vi "Version_2.0_Single_Column_Code.vi"() -> ()   [LabVIEW 2020] (continued)
                                n2523 = case shown="\"Standard Pumping\", Default" w2963 {
                                tunnel: w2965 -> [w2970 w2979]
                                tunnel: w2961 -> [w2971 w2978]
                                tunnel: [w2969 w2976] -> w2960
                                tunnel: w2962 -> [w2968 w2977]
                                frame "Standard Pumping", Default {
                                n2524 = Subtract(x=w2970, y=w2971) -> (x-y=w2967:dbl)
                                n2525 = Absolute Value(x=w2967) -> (abs(x)=w2966:dbl)
                                n2526 = Multiply(x=w2966, y=w2968) -> (x*y=w2973:dbl)
                                n2527 = Divide(x=w2973, y=3000.0) -> (x/y=w2969:dbl)
                                }
                                frame "High Resolution Pumping" {
                                n2528 = Subtract(x=w2979, y=w2978) -> (x-y=w2975:dbl)
                                n2529 = Absolute Value(x=w2975) -> (abs(x)=w2974:dbl)
                                n2530 = Multiply(x=w2974, y=w2977) -> (x*y=w2981:dbl)
                                n2531 = Divide(x=w2981, y=24000.0) -> (x/y=w2976:dbl)
                                }
                                }
                                n2532 = local write "Volume being Injected \nin this process"(w2960) -> ()
                                }
                                frame #1 {
                                n2533 = local read "Stopper that ends \nthe main loops"() -> (w2982:bool)
                                n2534 = call "LSPOneStatus (SubVI).vi"("VISA Refnum in"=w2985) -> ("read buffer"=w2987:string)  [unwired: 10 in]
                                n2535 = call <vilib>:"Trim Whitespace.vi"("string"=w2987) -> ("trimmed string"=w2986:string)  [unwired: 1 in]
                                n2536 = Equal?(x=w2986, y="/0`\u0003") -> (x = y?=w2984:bool)
                                n2537 = Or(x=w2984, y=w2982) -> (x .or. y?=w2983:bool)
                                }
                                }
                                n2538 = Wait (ms)(milliseconds to wait=u32 100) -> ()  [unwired: 1 out]
                                n2539 = local read "Stopper that ends \nthe main loops"() -> (w2952:bool)
                                n2540 = case shown="True" w2952 {
                                frame False {
                                }
                                frame True {
                                n2541 = local read "VISA Refnum in\nfor Pump"() -> (w2959:refnum<visa-resource-name>)
                                n2542 = call "HardStopCurrentProcess (SubVI).vi"("VISA Refnum in"=w2959) -> ()  [unwired: 11 in]
                                }
                                }
                                }
                                }
                                frame #11 {
                                # "Change the pump port back to Buffer-C1"
                                n2543 = local read "VISA Refnum in\nfor Pump"() -> (w2990:refnum<visa-resource-name>)
                                n2544 = local read "Port for \nC1-Equilibriation"() -> (w2989:string)
                                n2545 = local write "Pause Data Collection"(TRUE ("Pause Data Collection")) -> ()
                                n2546 = Wait (ms)(milliseconds to wait=u32 500) -> ()  [unwired: 1 out]
                                n2547 = call "PortChanger (SubVI).vi"("Port Number"=w2989, "VISA Refnum in"=w2990) -> ()  [unwired: 10 in]
                                }
                                frame #12 {
                                n2548 = local read "VISA Refnum in\nfor Pump"() -> (w2993:refnum<visa-resource-name>)
                                n2549 = local write "Volume being Injected \nin this process"(0.0 ("Volume being Injected \nin this process")) -> ()
                                n2550 = call "ProcessCompletionWaiter (SubVI).vi"("VISA Refnum in"=w2993) -> ()  [unwired: 11 in]
                                }
                              }
                            }
                            n2551 = local write "Reminder of the \nVolume to be \nPumped"(w2856) -> ()
                          }
                          frame #9 {
                            n2552 = stacked-sequence {
                              frame #0 {
                                n2553 = local read "Buffer-C1 PickUp \nFlow Rate (ul/min)\nfor Equilibration \nof Column-2"() -> (w2997:dbl)
                                n2554 = local read "Buffer-C1 Pumping\nResolution \nfor Equilibration \nof Column-2"() -> (w2996:T2)
                                n2555 = local read "VISA Refnum in\nfor Pump"() -> (w2999:refnum<visa-resource-name>)
                                n2556 = local read "Reminder of the \nVolume to be \nPumped"() -> (w2995:dbl)
                                n2557 = local read "Volume of Syringe"() -> (w2998:dbl)
                                n2558 = call "RPickUp(SubVI).vi"("Volume to be picked up"=w2995, "Volume of Syringe"=w2998, "Resolution of PickUP"=w2996, "PickUp Flow Rate (ul/min)"=w2997, "VISA Refnum in"=w2999) -> ()  [unwired: 6 in, 1 out]
                              }
                              frame #1 {
                                n2559 = while {
                                stop <- w3000 stop-if-true
                                n2560 = local read "Stopper that ends \nthe main loops"() -> (w3001:bool)
                                n2561 = local read "VISA Refnum in\nfor Pump"() -> (w3002:refnum<visa-resource-name>)
                                n2562 = case shown="True" w3001 {
                                frame False {
                                }
                                frame True {
                                n2563 = local read "VISA Refnum in\nfor Pump"() -> (w3003:refnum<visa-resource-name>)
                                n2564 = call "HardStopCurrentProcess (SubVI).vi"("VISA Refnum in"=w3003) -> ()  [unwired: 11 in]
                                }
                                }
                                n2565 = call "ProcessCompletionWaiterWithOutPut (SubVI).vi"("VISA Refnum in"=w3002) -> ("Boolean"=w3000:bool)  [unwired: 10 in]
                                }
                              }
                              frame #2 {
                                # "Reads the initial Plunger Position for computing the volume dispensed"
                                n2566 = local read "VISA Refnum in\nfor Pump"() -> (w3005:refnum<visa-resource-name>)
                                n2567 = call "AbsolutePlungerPosition (SubVI).vi"("VISA Refnum in"=w3005) -> ("Plunger Position"=w3004:i32)  [unwired: 10 in]
                                n2568 = local write "Initial Plunger Position"(w3004) -> ()
                              }
                              frame #3 {
                                # "Switch to Port-10"
                                # "Port-10 of the pump is conncted to column-2 of chip"
                                n2569 = local read "VISA Refnum in\nfor Pump"() -> (w3007:refnum<visa-resource-name>)
                                n2570 = call "PortChanger (SubVI).vi"("Port Number"="10", "VISA Refnum in"=w3007) -> ()  [unwired: 10 in]
                              }
                              frame #4 {
                                n2571 = while {
                                stop <- w3008 stop-if-true
                                n2572 = local read "Stopper that ends \nthe main loops"() -> (w3009:bool)
                                n2573 = local read "VISA Refnum in\nfor Pump"() -> (w3010:refnum<visa-resource-name>)
                                n2574 = case shown="True" w3009 {
                                frame False {
                                }
                                frame True {
                                n2575 = local read "VISA Refnum in\nfor Pump"() -> (w3011:refnum<visa-resource-name>)
                                n2576 = call "HardStopCurrentProcess (SubVI).vi"("VISA Refnum in"=w3011) -> ()  [unwired: 11 in]
                                }
                                }
                                n2577 = call "ProcessCompletionWaiterWithOutPut (SubVI).vi"("VISA Refnum in"=w3010) -> ("Boolean"=w3008:bool)  [unwired: 10 in]
                                }
                              }
                              frame #5 {
                                # "Keeps the AMF valve after column-1 open and valve after column-2 closed"
                                n2578 = local read "Buffer-C1 Dispense\nFlow Rate (ul/min) \nfor Equilibration\nof Column-2"() -> (w3024:dbl)
                                n2579 = local read "Buffer-C1 Pumping\nResolution \nfor Equilibration \nof Column-2"() -> (w3023:T2)
                                n2580 = local read "VISA Refnum in\nfor Pump"() -> (w3026:refnum<visa-resource-name>)
                                n2581 = local write "Pause Data Collection"(FALSE ("Pause Data Collection")) -> ()
                                n2582 = local read "Volume of Syringe"() -> (w3025:dbl)
                                n2583 = call "GoToAbsolutePosition(SubVI).vi"("Absolute Volume Position in Syringe (in ul)"=0.0, "Volume of Syringe"=w3025, "Resolution of Pumping"=w3023, "Flow Rate (ul/min)"=w3024, "VISA Refnum in"=w3026) -> ()  [unwired: 6 in, 1 out]
                                n2584 = local read "VISA Refnum in\nfor Valve"() -> (w3016:refnum<visa-resource-name>)
                                n2585 = local write "Valve V1 Open"(FALSE ("Valve V1 Open")) -> ()
                                n2586 = local write "Valve V2 Open"(TRUE ("Valve V2 Open")) -> ()
                                n2587 = local write "Valve V3 Open"(TRUE ("Valve V3 Open")) -> ()
                                n2588 = local write "Valve V4 Open"(FALSE ("Affinity On")) -> ()
                                n2589 = local read "External Valve \nOPEN"() -> (w3015:string)
                                n2590 = local write "Valve V5 Open"(FALSE ("Valve V5 Open")) -> ()
                                n2591 = local write "Valve V6 Open"(FALSE ("Valve V6 Open")) -> ()
                                n2592 = local write "Valve V7 Open"(FALSE ("Valve V7 Open")) -> ()
                                n2593 = call "PortChanger_Valve (SubVI).vi"("Port Number"=w3015, "VISA Refnum in"=w3016) -> ()  [unwired: 10 in]
                              }
                              frame #6 {
                                n2594 = local read "Buffer-C1 Pumping\nResolution \nfor Equilibration \nof Column-2"() -> (w3028:T2)
                                n2595 = local read "VISA Refnum in\nfor Pump"() -> (w3030:refnum<visa-resource-name>)
                                n2596 = local read "Initial Plunger Position"() -> (w3029:dbl)
                                n2597 = local read "Volume of Syringe"() -> (w3027:dbl)
                                n2598 = while {
                                tunnel: w3029 -> [w3037]
                                tunnel: w3030 -> [w3036]
                                tunnel: w3028 -> [w3035]
                                tunnel: w3027 -> [w3034]
                                stop <- w3032 stop-if-true
                                n2599 = stacked-sequence {
                                tunnel: w3037 -> [w3044 _]
                                tunnel: w3036 -> [w3043 w3068]
                                tunnel: w3035 -> [w3042 _]
                                tunnel: w3034 -> [w3041 _]
                                tunnel: [_ w3066] -> w3032
                                frame #0 {
                                n2600 = call "AbsolutePlungerPosition (SubVI).vi"("VISA Refnum in"=w3043) -> ("Plunger Position"=w3040:i32)  [unwired: 10 in]
                                n2601 = case shown="\"Standard Pumping\", Default" w3042 {
                                tunnel: w3044 -> [w3049 w3058]
                                tunnel: w3040 -> [w3050 w3057]
                                tunnel: [w3048 w3055] -> w3039
                                tunnel: w3041 -> [w3047 w3056]
                                frame "Standard Pumping", Default {
                                n2602 = Subtract(x=w3049, y=w3050) -> (x-y=w3046:dbl)
                                n2603 = Absolute Value(x=w3046) -> (abs(x)=w3045:dbl)
                                n2604 = Multiply(x=w3045, y=w3047) -> (x*y=w3052:dbl)
                                n2605 = Divide(x=w3052, y=3000.0) -> (x/y=w3048:dbl)
                                }
                                frame "High Resolution Pumping" {
                                n2606 = Subtract(x=w3058, y=w3057) -> (x-y=w3054:dbl)
                                n2607 = Absolute Value(x=w3054) -> (abs(x)=w3053:dbl)
                                n2608 = Multiply(x=w3053, y=w3056) -> (x*y=w3060:dbl)
                                n2609 = Divide(x=w3060, y=24000.0) -> (x/y=w3055:dbl)
                                }
                                }
                                n2610 = local write "Volume being Injected \nin this process"(w3039) -> ()
                                }
                                frame #1 {
                                n2611 = local read "Buffer-C Volume \nto be Pumped for\nColumn \nnon-interference"() -> (w3064:dbl)
                                n2612 = local read "Volume being Injected \nin this process"() -> (w3065:dbl)
                                n2613 = local read "Stopper that ends \nthe main loops"() -> (w3063:bool)
                                n2614 = call "LSPOneStatus (SubVI).vi"("VISA Refnum in"=w3068) -> ("read buffer"=w3070:string)  [unwired: 10 in]
                                n2615 = call <vilib>:"Trim Whitespace.vi"("string"=w3070) -> ("trimmed string"=w3069:string)  [unwired: 1 in]
                                n2616 = Equal?(x=w3069, y="/0`\u0003") -> (x = y?=w3067:bool)
                                n2617 = Greater Or Equal?(x=w3065, y=w3064) -> (x >= y?=w3062:bool)
                                n2618 = Or(x=w3063, y=w3062) -> (x .or. y?=w3061:bool)
                                n2619 = Or(x=w3067, y=w3061) -> (x .or. y?=w3066:bool)
                                }
                                }
                                n2620 = Wait (ms)(milliseconds to wait=u32 100) -> ()  [unwired: 1 out]
                                n2621 = local read "Stopper that ends \nthe main loops"() -> (w3031:bool)
                                n2622 = case shown="True" w3031 {
                                frame False {
                                }
                                frame True {
                                n2623 = local read "VISA Refnum in\nfor Pump"() -> (w3038:refnum<visa-resource-name>)
                                n2624 = call "HardStopCurrentProcess (SubVI).vi"("VISA Refnum in"=w3038) -> ()  [unwired: 11 in]
                                }
                                }
                                }
                              }
                              frame #7 {
                                # "Keeps the AMF valve after column-1 closed and valve after column-2 open"
                                n2625 = local read "VISA Refnum in\nfor Valve"() -> (w3076:refnum<visa-resource-name>)
                                n2626 = local read "External Valve \nCLOSED"() -> (w3075:string)
                                n2627 = local write "Valve V4 Open"(TRUE ("Valve V4 Open")) -> ()
                                n2628 = local write "Valve V1 Open"(FALSE ("Valve V1 Open")) -> ()
                                n2629 = local write "Valve V2 Open"(FALSE ("Valve V2 Open")) -> ()
                                n2630 = local write "Valve V3 Open"(FALSE ("Valve V3 Open")) -> ()
                                n2631 = call "PortChanger_Valve (SubVI).vi"("Port Number"=w3075, "VISA Refnum in"=w3076) -> ()  [unwired: 10 in]
                                n2632 = local write "Valve V7 Open"(TRUE ("Valve V7 Open")) -> ()
                                n2633 = local write "Valve V5 Open"(TRUE ("Valve V5 Open")) -> ()
                                n2634 = local write "Valve V6 Open"(TRUE ("Valve V6 Open")) -> ()
                              }
                              frame #8 {
                                n2635 = local read "Buffer-C1 Pumping\nResolution \nfor Equilibration \nof Column-2"() -> (w3082:T2)
                                n2636 = local read "VISA Refnum in\nfor Pump"() -> (w3084:refnum<visa-resource-name>)
                                n2637 = local read "Initial Plunger Position"() -> (w3083:dbl)
                                n2638 = local read "Volume of Syringe"() -> (w3081:dbl)
                                n2639 = while {
                                tunnel: w3083 -> [w3091]
                                tunnel: w3084 -> [w3090]
                                tunnel: w3082 -> [w3089]
                                tunnel: w3081 -> [w3088]
                                stop <- w3086 stop-if-true
                                n2640 = stacked-sequence {
                                tunnel: w3091 -> [w3098 _]
                                tunnel: w3090 -> [w3097 w3118]
                                tunnel: w3089 -> [w3096 _]
                                tunnel: w3088 -> [w3095 _]
                                tunnel: [_ w3116] -> w3086
                                frame #0 {
                                n2641 = call "AbsolutePlungerPosition (SubVI).vi"("VISA Refnum in"=w3097) -> ("Plunger Position"=w3094:i32)  [unwired: 10 in]
                                n2642 = case shown="\"Standard Pumping\", Default" w3096 {
                                tunnel: w3098 -> [w3103 w3112]
                                tunnel: w3094 -> [w3104 w3111]
                                tunnel: [w3102 w3109] -> w3093
                                tunnel: w3095 -> [w3101 w3110]
                                frame "Standard Pumping", Default {
                                n2643 = Subtract(x=w3103, y=w3104) -> (x-y=w3100:dbl)
                                n2644 = Absolute Value(x=w3100) -> (abs(x)=w3099:dbl)
                                n2645 = Multiply(x=w3099, y=w3101) -> (x*y=w3106:dbl)
                                n2646 = Divide(x=w3106, y=3000.0) -> (x/y=w3102:dbl)
                                }
                                frame "High Resolution Pumping" {
                                n2647 = Subtract(x=w3112, y=w3111) -> (x-y=w3108:dbl)
                                n2648 = Absolute Value(x=w3108) -> (abs(x)=w3107:dbl)
                                n2649 = Multiply(x=w3107, y=w3110) -> (x*y=w3114:dbl)
                                n2650 = Divide(x=w3114, y=24000.0) -> (x/y=w3109:dbl)
                                }
                                }
                                n2651 = local write "Volume being Injected \nin this process"(w3093) -> ()
                                }
                                frame #1 {
                                n2652 = local read "Stopper that ends \nthe main loops"() -> (w3115:bool)
                                n2653 = call "LSPOneStatus (SubVI).vi"("VISA Refnum in"=w3118) -> ("read buffer"=w3120:string)  [unwired: 10 in]
                                n2654 = call <vilib>:"Trim Whitespace.vi"("string"=w3120) -> ("trimmed string"=w3119:string)  [unwired: 1 in]
                                n2655 = Equal?(x=w3119, y="/0`\u0003") -> (x = y?=w3117:bool)
                                n2656 = Or(x=w3117, y=w3115) -> (x .or. y?=w3116:bool)
                                }
                                }
                                n2657 = Wait (ms)(milliseconds to wait=u32 100) -> ()  [unwired: 1 out]
                                n2658 = local read "Stopper that ends \nthe main loops"() -> (w3085:bool)
                                n2659 = case shown="True" w3085 {
                                frame False {
                                }
                                frame True {
                                n2660 = local read "VISA Refnum in\nfor Pump"() -> (w3092:refnum<visa-resource-name>)
                                n2661 = call "HardStopCurrentProcess (SubVI).vi"("VISA Refnum in"=w3092) -> ()  [unwired: 11 in]
                                }
                                }
                                }
                              }
                              frame #9 {
                                n2662 = local write "Pause Data Collection"(TRUE ("Pause Data Collection")) -> ()
                                n2663 = Wait (ms)(milliseconds to wait=u32 500) -> ()  [unwired: 1 out]
                              }
                              frame #10 {
                                n2664 = local write "Volume being Injected \nin this process"(0.0 ("Volume being Injected \nin this process")) -> ()
                                n2665 = local write "Start the Process"(FALSE ("Start the Process")) -> ()
                              }
                            }
                          }
                          frame #10 {
                            # "Clean the tubing with Sample"
                            n2666 = local read "N-S"() -> (w3126:i32)
                            n2667 = for {
                              N: w3126 -> [_]
                              n2668 = stacked-sequence {
                                frame #0 {
                                n2669 = local read "VISA Refnum in\nfor Pump"() -> (w3129:refnum<visa-resource-name>)
                                n2670 = local read "Port for \nSample"() -> (w3128:string)
                                n2671 = call "PortChanger (SubVI).vi"("Port Number"=w3128, "VISA Refnum in"=w3129) -> ()  [unwired: 10 in]
                                }
                                frame #1 {
                                n2672 = local read "VISA Refnum in\nfor Pump"() -> (w3130:refnum<visa-resource-name>)
                                n2673 = call "ProcessCompletionWaiter (SubVI).vi"("VISA Refnum in"=w3130) -> ()  [unwired: 11 in]
                                }
                                frame #2 {
                                n2674 = local read "VISA Refnum in\nfor Pump"() -> (w3135:refnum<visa-resource-name>)
                                n2675 = local read "Sample PickUp \nFlow Rate (ul/min)"() -> (w3132:dbl)
                                n2676 = local read "V-S"() -> (w3131:dbl)
                                n2677 = local read "Volume of Syringe"() -> (w3133:dbl)
                                n2678 = call "RPickUp(SubVI).vi"("Volume to be picked up"=w3131, "Volume of Syringe"=w3133, "Resolution of PickUP"=T2."Standard Pumping", "PickUp Flow Rate (ul/min)"=w3132, "VISA Refnum in"=w3135) -> ()  [unwired: 6 in, 1 out]
                                }
                                frame #3 {
                                n2679 = local read "Stopper that ends \nthe main loops"() -> (w3136:bool)
                                n2680 = local read "VISA Refnum in\nfor Pump"() -> (w3137:refnum<visa-resource-name>)
                                n2681 = case shown="True" w3136 {
                                frame False {
                                }
                                frame True {
                                n2682 = local read "VISA Refnum in\nfor Pump"() -> (w3138:refnum<visa-resource-name>)
                                n2683 = call "HardStopCurrentProcess (SubVI).vi"("VISA Refnum in"=w3138) -> ()  [unwired: 11 in]
                                }
                                }
                                n2684 = call "ProcessCompletionWaiter (SubVI).vi"("VISA Refnum in"=w3137) -> ()  [unwired: 11 in]
                                }
                                frame #4 {
                                n2685 = local read "VISA Refnum in\nfor Pump"() -> (w3140:refnum<visa-resource-name>)
                                n2686 = call "PortChanger (SubVI).vi"("Port Number"="1", "VISA Refnum in"=w3140) -> ()  [unwired: 10 in]
                                }
                                frame #5 {
                                n2687 = local read "Stopper that ends \nthe main loops"() -> (w3141:bool)
                                n2688 = local read "VISA Refnum in\nfor Pump"() -> (w3142:refnum<visa-resource-name>)
                                n2689 = case shown="True" w3141 {
                                frame False {
                                }
                                frame True {
                                n2690 = local read "VISA Refnum in\nfor Pump"() -> (w3143:refnum<visa-resource-name>)
                                n2691 = call "HardStopCurrentProcess (SubVI).vi"("VISA Refnum in"=w3143) -> ()  [unwired: 11 in]
                                }
                                }
                                n2692 = call "ProcessCompletionWaiter (SubVI).vi"("VISA Refnum in"=w3142) -> ()  [unwired: 11 in]
                                }
                                frame #6 {
                                n2693 = local read "VISA Refnum in\nfor Pump"() -> (w3148:refnum<visa-resource-name>)
                                n2694 = local read "Volume of Syringe"() -> (w3145:dbl)
                                n2695 = call "GoToAbsolutePosition(SubVI).vi"("Absolute Volume Position in Syringe (in ul)"=0.0 ("Volume to be picked up"), "Volume of Syringe"=w3145, "Resolution of Pumping"=T2."Standard Pumping" ("Resolution of PickUP"), "Flow Rate (ul/min)"=150.0 ("PickUp Flow Rate (ul/min)"), "VISA Refnum in"=w3148) -> ()  [unwired: 6 in, 1 out]
                                }
                                frame #7 {
                                n2696 = local read "Stopper that ends \nthe main loops"() -> (w3149:bool)
                                n2697 = local read "VISA Refnum in\nfor Pump"() -> (w3150:refnum<visa-resource-name>)
                                n2698 = case shown="True" w3149 {
                                frame False {
                                }
                                frame True {
                                n2699 = local read "VISA Refnum in\nfor Pump"() -> (w3151:refnum<visa-resource-name>)
                                n2700 = call "HardStopCurrentProcess (SubVI).vi"("VISA Refnum in"=w3151) -> ()  [unwired: 11 in]
                                }
                                }
                                n2701 = call "ProcessCompletionWaiter (SubVI).vi"("VISA Refnum in"=w3150) -> ()  [unwired: 11 in]
                                }
                              }
                              n2702 = local write "Pause Data Collection"(TRUE ("Pause Data Collection")) -> ()
                            }
                          }
                        }
                      }
                      frame #1 {
                        # "Pump Purified Sample into Column-2"
                        n2703 = stacked-sequence {
                          frame #0 {
                            # "Switch to Port-3"
                            # "Port-3 of pump is connected to Sample"
                            n2704 = local read "VISA Refnum in\nfor Pump"() -> (w3156:refnum<visa-resource-name>)
                            n2705 = local read "Port for \nSample"() -> (w3155:string)
                            n2706 = call "PortChanger (SubVI).vi"("Port Number"=w3155, "VISA Refnum in"=w3156) -> ()  [unwired: 10 in]
                          }
                          frame #1 {
                            n2707 = local read "VISA Refnum in\nfor Pump"() -> (w3157:refnum<visa-resource-name>)
                            n2708 = call "ProcessCompletionWaiter (SubVI).vi"("VISA Refnum in"=w3157) -> ()  [unwired: 11 in]
                          }
                          frame #2 {
                            # "V4 is open"
                            # "V1, V2 and V3 are closed"
                            n2709 = local read "VISA Refnum in\nfor Valve"() -> (w3162:refnum<visa-resource-name>)
                            n2710 = local read "External Valve \nCLOSED"() -> (w3161:string)
                            n2711 = local write "Valve V1 Open"(FALSE ("Valve V1 Open")) -> ()
                            n2712 = local write "Valve V2 Open"(FALSE ("Valve V2 Open")) -> ()
                            n2713 = local write "Valve V3 Open"(FALSE ("Valve V3 Open")) -> ()
                            n2714 = local write "Valve V4 Open"(TRUE ("Valve V4 Open")) -> ()
                            n2715 = call "PortChanger_Valve (SubVI).vi"("Port Number"=w3161, "VISA Refnum in"=w3162) -> ()  [unwired: 10 in]
                            n2716 = local write "Valve V5 Open"(TRUE ("Valve V5 Open")) -> ()
                            n2717 = local write "Valve V6 Open"(TRUE ("Valve V6 Open")) -> ()
                            n2718 = local write "Valve V7 Open"(FALSE ("Valve V7 Open")) -> ()
                          }
                          frame #3 {
                            n2719 = local read "Apparent Volume\nof Syringe"() -> (w3167:dbl)
                            n2720 = local read "Sample Volume \nto be Pumped"() -> (w3170:dbl)
                            n2721 = Quotient & Remainder(x=w3170, y=w3167) -> (x-y*floor(x/y)=w3168:dbl, floor(x/y)=w3169:dbl)
                            n2722 = for {
                              N: w3169 -> [_]
                              n2723 = stacked-sequence {
                                frame #0 {
                                n2724 = local read "Sample PickUp \nFlow Rate (ul/min)"() -> (w3173:dbl)
                                n2725 = local read "Sample Pumping\nResolution"() -> (w3172:T2)
                                n2726 = local read "VISA Refnum in\nfor Pump"() -> (w3175:refnum<visa-resource-name>)
                                n2727 = local read "Apparent Volume\nof Syringe"() -> (w3171:dbl)
                                n2728 = local read "Volume of Syringe"() -> (w3174:dbl)
                                n2729 = call "RPickUp(SubVI).vi"("Volume to be picked up"=w3171, "Volume of Syringe"=w3174, "Resolution of PickUP"=w3172, "PickUp Flow Rate (ul/min)"=w3173, "VISA Refnum in"=w3175) -> ()  [unwired: 6 in, 1 out]
                                }
                                frame #1 {
                                n2730 = local read "Stopper that ends \nthe main loops"() -> (w3176:bool)
                                n2731 = local read "VISA Refnum in\nfor Pump"() -> (w3177:refnum<visa-resource-name>)
                                n2732 = case shown="True" w3176 {
                                frame False {
                                }
                                frame True {
                                n2733 = local read "VISA Refnum in\nfor Pump"() -> (w3178:refnum<visa-resource-name>)
                                n2734 = call "HardStopCurrentProcess (SubVI).vi"("VISA Refnum in"=w3178) -> ()  [unwired: 11 in]
                                }
                                }
                                n2735 = call "ProcessCompletionWaiter (SubVI).vi"("VISA Refnum in"=w3177) -> ()  [unwired: 11 in]
                                }
                                frame #2 {
                                # "Reads the initial Plunger Position for computing the volume dispensed"
                                n2736 = local read "VISA Refnum in\nfor Pump"() -> (w3180:refnum<visa-resource-name>)
                                n2737 = call "AbsolutePlungerPosition (SubVI).vi"("VISA Refnum in"=w3180) -> ("Plunger Position"=w3179:i32)  [unwired: 10 in]
                                n2738 = local write "Initial Plunger Position"(w3179) -> ()
                                }
                                frame #3 {
                                # "Switch to Port-2"
                                # "Port-2 of the pump is conncted to column-1 of chip"
                                n2739 = local read "VISA Refnum in\nfor Pump"() -> (w3182:refnum<visa-resource-name>)
                                n2740 = call "PortChanger (SubVI).vi"("Port Number"="10", "VISA Refnum in"=w3182) -> ()  [unwired: 10 in]
                                }
                                frame #4 {
                                n2741 = local read "Stopper that ends \nthe main loops"() -> (w3183:bool)
                                n2742 = local read "VISA Refnum in\nfor Pump"() -> (w3184:refnum<visa-resource-name>)
                                n2743 = case shown="True" w3183 {
                                frame False {
                                }
                                frame True {
                                n2744 = local read "VISA Refnum in\nfor Pump"() -> (w3185:refnum<visa-resource-name>)
                                n2745 = call "HardStopCurrentProcess (SubVI).vi"("VISA Refnum in"=w3185) -> ()  [unwired: 11 in]
                                }
                                }
                                n2746 = call "ProcessCompletionWaiter (SubVI).vi"("VISA Refnum in"=w3184) -> ()  [unwired: 11 in]
                                }
                                frame #5 {
                                # "Keeps the AMF valve after column-1 open and valve after column-2 closed"
                                n2747 = local read "Sample Dispense\nFlow Rate (ul/min)"() -> (w3189:dbl)
                                n2748 = local read "Sample Pumping\nResolution"() -> (w3188:T2)
                                n2749 = local read "VISA Refnum in\nfor Pump"() -> (w3191:refnum<visa-resource-name>)
                                n2750 = local write "Pause Data Collection"(FALSE ("Pause Data Collection")) -> ()
                                n2751 = local read "Volume of Syringe"() -> (w3190:dbl)
                                n2752 = call "GoToAbsolutePosition(SubVI).vi"("Absolute Volume Position in Syringe (in ul)"=0.0 ("Volume to be Dispensed"), "Volume of Syringe"=w3190, "Resolution of Pumping"=w3188, "Flow Rate (ul/min)"=w3189, "VISA Refnum in"=w3191) -> ()  [unwired: 6 in, 1 out]
                                }
                                frame #6 {
                                n2753 = local read "Sample Pumping\nResolution"() -> (w3193:T2)
                                n2754 = local read "VISA Refnum in\nfor Pump"() -> (w3195:refnum<visa-resource-name>)
                                n2755 = local read "Initial Plunger Position"() -> (w3194:dbl)
                                n2756 = local read "Volume of Syringe"() -> (w3192:dbl)
                                n2757 = while {
                                tunnel: w3194 -> [w3202]
                                tunnel: w3195 -> [w3201]
                                tunnel: w3193 -> [w3200]
                                tunnel: w3192 -> [w3199]
                                stop <- w3197 stop-if-true
                                n2758 = stacked-sequence {
                                tunnel: w3202 -> [w3209 _]
                                tunnel: w3201 -> [w3208 w3229]
                                tunnel: w3200 -> [w3207 _]
                                tunnel: w3199 -> [w3206 _]
                                tunnel: [_ w3227] -> w3197
                                frame #0 {
                                n2759 = call "AbsolutePlungerPosition (SubVI).vi"("VISA Refnum in"=w3208) -> ("Plunger Position"=w3205:i32)  [unwired: 10 in]
                                n2760 = case shown="\"Standard Pumping\", Default" w3207 {
                                tunnel: w3209 -> [w3214 w3223]
                                tunnel: w3205 -> [w3215 w3222]
                                tunnel: [w3213 w3220] -> w3204
                                tunnel: w3206 -> [w3212 w3221]
                                frame "Standard Pumping", Default {
                                n2761 = Subtract(x=w3214, y=w3215) -> (x-y=w3211:dbl)
                                n2762 = Absolute Value(x=w3211) -> (abs(x)=w3210:dbl)
                                n2763 = Multiply(x=w3210, y=w3212) -> (x*y=w3217:dbl)
                                n2764 = Divide(x=w3217, y=3000.0) -> (x/y=w3213:dbl)
                                }
                                frame "High Resolution Pumping" {
                                n2765 = Subtract(x=w3223, y=w3222) -> (x-y=w3219:dbl)
                                n2766 = Absolute Value(x=w3219) -> (abs(x)=w3218:dbl)
                                n2767 = Multiply(x=w3218, y=w3221) -> (x*y=w3225:dbl)
                                n2768 = Divide(x=w3225, y=24000.0) -> (x/y=w3220:dbl)
                                }
                                }
                                n2769 = local write "Volume being Injected \nin this process"(w3204) -> ()
                                }
                                frame #1 {
                                n2770 = call "LSPOneStatus (SubVI).vi"("VISA Refnum in"=w3229) -> ("read buffer"=w3231:string)  [unwired: 10 in]
                                n2771 = call <vilib>:"Trim Whitespace.vi"("string"=w3231) -> ("trimmed string"=w3230:string)  [unwired: 1 in]
                                n2772 = local read "Stopper that ends \nthe main loops"() -> (w3226:bool)
                                n2773 = Equal?(x=w3230, y="/0`\u0003") -> (x = y?=w3228:bool)
                                n2774 = Or(x=w3228, y=w3226) -> (x .or. y?=w3227:bool)
                                }
                                }
                                n2775 = Wait (ms)(milliseconds to wait=u32 100) -> ()  [unwired: 1 out]
                                n2776 = local read "Stopper that ends \nthe main loops"() -> (w3196:bool)
                                n2777 = case shown="True" w3196 {
                                frame False {
                                }
                                frame True {
                                n2778 = local read "VISA Refnum in\nfor Pump"() -> (w3203:refnum<visa-resource-name>)
                                n2779 = call "HardStopCurrentProcess (SubVI).vi"("VISA Refnum in"=w3203) -> ()  [unwired: 11 in]
                                }
                                }
                                }
                                }
                                frame #7 {
                                # "Chnage the pump port back to Sample"
                                n2780 = local read "VISA Refnum in\nfor Pump"() -> (w3234:refnum<visa-resource-name>)
                                n2781 = local read "Port for \nSample"() -> (w3233:string)
                                n2782 = local write "Pause Data Collection"(TRUE ("Pause Data Collection")) -> ()
                                n2783 = Wait (ms)(milliseconds to wait=u32 500) -> ()  [unwired: 1 out]
                                n2784 = call "PortChanger (SubVI).vi"("Port Number"=w3233, "VISA Refnum in"=w3234) -> ()  [unwired: 10 in]
                                }
                                frame #8 {
                                n2785 = local read "VISA Refnum in\nfor Pump"() -> (w3237:refnum<visa-resource-name>)
                                n2786 = local write "Volume being Injected \nin this process"(0.0 ("Volume being Injected \nin this process")) -> ()
                                n2787 = call "ProcessCompletionWaiter (SubVI).vi"("VISA Refnum in"=w3237) -> ()  [unwired: 11 in]
                                }
                              }
                            }
                            n2788 = local write "Reminder of the \nVolume to be \nPumped"(w3168) -> ()
                          }
                          frame #4 {
                            n2789 = stacked-sequence {
                              frame #0 {
                                n2790 = local read "Sample PickUp \nFlow Rate (ul/min)"() -> (w3241:dbl)
                                n2791 = local read "Sample Pumping\nResolution"() -> (w3240:T2)
                                n2792 = local read "VISA Refnum in\nfor Pump"() -> (w3243:refnum<visa-resource-name>)
                                n2793 = local read "Reminder of the \nVolume to be \nPumped"() -> (w3239:dbl)
                                n2794 = local read "Volume of Syringe"() -> (w3242:dbl)
                                n2795 = call "RPickUp(SubVI).vi"("Volume to be picked up"=w3239, "Volume of Syringe"=w3242, "Resolution of PickUP"=w3240, "PickUp Flow Rate (ul/min)"=w3241, "VISA Refnum in"=w3243) -> ()  [unwired: 6 in, 1 out]
                              }
                              frame #1 {
                                n2796 = local read "Stopper that ends \nthe main loops"() -> (w3244:bool)
                                n2797 = local read "VISA Refnum in\nfor Pump"() -> (w3245:refnum<visa-resource-name>)
                                n2798 = case shown="True" w3244 {
                                frame False {
                                }
                                frame True {
                                n2799 = local read "VISA Refnum in\nfor Pump"() -> (w3246:refnum<visa-resource-name>)
                                n2800 = call "HardStopCurrentProcess (SubVI).vi"("VISA Refnum in"=w3246) -> ()  [unwired: 11 in]
                                }
                                }
                                n2801 = call "ProcessCompletionWaiter (SubVI).vi"("VISA Refnum in"=w3245) -> ()  [unwired: 11 in]
                              }
                              frame #2 {
                                # "Reads the initial Plunger Position for computing the volume dispensed"
                                n2802 = local read "VISA Refnum in\nfor Pump"() -> (w3248:refnum<visa-resource-name>)
                                n2803 = call "AbsolutePlungerPosition (SubVI).vi"("VISA Refnum in"=w3248) -> ("Plunger Position"=w3247:i32)  [unwired: 10 in]
                                n2804 = local write "Initial Plunger Position"(w3247) -> ()
                              }
                              frame #3 {
                                # "Switch to Port-2"
                                # "Port-2 of the pump is conncted to column-1 of chip"
                                n2805 = local read "VISA Refnum in\nfor Pump"() -> (w3250:refnum<visa-resource-name>)
                                n2806 = call "PortChanger (SubVI).vi"("Port Number"="10", "VISA Refnum in"=w3250) -> ()  [unwired: 10 in]
                              }
                              frame #4 {
                                n2807 = local read "Stopper that ends \nthe main loops"() -> (w3251:bool)
                                n2808 = local read "VISA Refnum in\nfor Pump"() -> (w3252:refnum<visa-resource-name>)
                                n2809 = case shown="True" w3251 {
                                frame False {
                                }
                                frame True {
                                n2810 = local read "VISA Refnum in\nfor Pump"() -> (w3253:refnum<visa-resource-name>)
                                n2811 = call "HardStopCurrentProcess (SubVI).vi"("VISA Refnum in"=w3253) -> ()  [unwired: 11 in]
                                }
                                }
                                n2812 = call "ProcessCompletionWaiter (SubVI).vi"("VISA Refnum in"=w3252) -> ()  [unwired: 11 in]
                              }
                              frame #5 {
                                # "Keeps the AMF valve after column-1 open and valve after column-2 closed"
                                n2813 = local read "Sample Dispense\nFlow Rate (ul/min)"() -> (w3257:dbl)
                                n2814 = local read "Sample Pumping\nResolution"() -> (w3256:T2)
                                n2815 = local read "VISA Refnum in\nfor Pump"() -> (w3259:refnum<visa-resource-name>)
                                n2816 = local write "Pause Data Collection"(FALSE ("Pause Data Collection")) -> ()
                                n2817 = local read "Volume of Syringe"() -> (w3258:dbl)
                                n2818 = call "GoToAbsolutePosition(SubVI).vi"("Absolute Volume Position in Syringe (in ul)"=0.0 ("Volume to be Dispensed"), "Volume of Syringe"=w3258, "Resolution of Pumping"=w3256, "Flow Rate (ul/min)"=w3257, "VISA Refnum in"=w3259) -> ()  [unwired: 6 in, 1 out]
                              }
                              frame #6 {
                                n2819 = local read "Sample Pumping\nResolution"() -> (w3261:T2)
                                n2820 = local read "VISA Refnum in\nfor Pump"() -> (w3263:refnum<visa-resource-name>)
                                n2821 = local read "Initial Plunger Position"() -> (w3262:dbl)
                                n2822 = local read "Volume of Syringe"() -> (w3260:dbl)
                                n2823 = while {
                                tunnel: w3262 -> [w3270]
                                tunnel: w3263 -> [w3269]
                                tunnel: w3261 -> [w3268]
                                tunnel: w3260 -> [w3267]
                                stop <- w3265 stop-if-true
                                n2824 = stacked-sequence {
                                tunnel: w3270 -> [w3277 _]
                                tunnel: w3269 -> [w3276 w3297]
                                tunnel: w3268 -> [w3275 _]
                                tunnel: w3267 -> [w3274 _]
                                tunnel: [_ w3295] -> w3265
                                frame #0 {
                                n2825 = call "AbsolutePlungerPosition (SubVI).vi"("VISA Refnum in"=w3276) -> ("Plunger Position"=w3273:i32)  [unwired: 10 in]
                                n2826 = case shown="\"Standard Pumping\", Default" w3275 {
                                tunnel: w3277 -> [w3282 w3291]
                                tunnel: w3273 -> [w3283 w3290]
                                tunnel: [w3281 w3288] -> w3272
                                tunnel: w3274 -> [w3280 w3289]
                                frame "Standard Pumping", Default {
                                n2827 = Subtract(x=w3282, y=w3283) -> (x-y=w3279:dbl)
                                n2828 = Absolute Value(x=w3279) -> (abs(x)=w3278:dbl)
                                n2829 = Multiply(x=w3278, y=w3280) -> (x*y=w3285:dbl)
                                n2830 = Divide(x=w3285, y=3000.0) -> (x/y=w3281:dbl)
                                }
                                frame "High Resolution Pumping" {
                                n2831 = Subtract(x=w3291, y=w3290) -> (x-y=w3287:dbl)
                                n2832 = Absolute Value(x=w3287) -> (abs(x)=w3286:dbl)
                                n2833 = Multiply(x=w3286, y=w3289) -> (x*y=w3293:dbl)
                                n2834 = Divide(x=w3293, y=24000.0) -> (x/y=w3288:dbl)
                                }
                                }
                                n2835 = local write "Volume being Injected \nin this process"(w3272) -> ()
                                }
                                frame #1 {
                                n2836 = call "LSPOneStatus (SubVI).vi"("VISA Refnum in"=w3297) -> ("read buffer"=w3299:string)  [unwired: 10 in]
                                n2837 = call <vilib>:"Trim Whitespace.vi"("string"=w3299) -> ("trimmed string"=w3298:string)  [unwired: 1 in]
                                n2838 = local read "Stopper that ends \nthe main loops"() -> (w3294:bool)
                                n2839 = Equal?(x=w3298, y="/0`\u0003") -> (x = y?=w3296:bool)
                                n2840 = Or(x=w3296, y=w3294) -> (x .or. y?=w3295:bool)
                                }
                                }
                                n2841 = Wait (ms)(milliseconds to wait=u32 100) -> ()  [unwired: 1 out]
                                n2842 = local read "Stopper that ends \nthe main loops"() -> (w3264:bool)
                                n2843 = case shown="True" w3264 {
                                frame False {
                                }
                                frame True {
                                n2844 = local read "VISA Refnum in\nfor Pump"() -> (w3271:refnum<visa-resource-name>)
                                n2845 = call "HardStopCurrentProcess (SubVI).vi"("VISA Refnum in"=w3271) -> ()  [unwired: 11 in]
                                }
                                }
                                }
                              }
                              frame #7 {
                                n2846 = local write "Pause Data Collection"(TRUE ("Pause Data Collection")) -> ()
                                n2847 = Wait (ms)(milliseconds to wait=u32 500) -> ()  [unwired: 1 out]
                              }
                              frame #8 {
                                n2848 = local write "Volume being Injected \nin this process"(0.0 ("Volume being Injected \nin this process")) -> ()
                              }
                            }
                          }
                        }
                        n2849 = local write "Equilibriating \nColumn-2"(FALSE ("Equilibriating \nColumn-2")) -> ()
                        n2850 = local write "Affinity On"(TRUE ("Affinity On")) -> ()
                        n2851 = local write "Sample pumping \ninto Column-1"(TRUE ("Sample pumping \ninto Column-1")) -> ()
                      }
                      frame #2 {
                        # "Wash Column-1 with Buffer-A2"
                        n2852 = stacked-sequence {
                          frame #0 {
                            # "Switch to Port-4/6"
                            # "Port-4/6 of pump is connected to Buffer-A2"
                            n2853 = local read "VISA Refnum in\nfor Pump"() -> (w3307:refnum<visa-resource-name>)
                            n2854 = local read "Port for \nA2-Wash"() -> (w3306:string)
                            n2855 = call "PortChanger (SubVI).vi"("Port Number"=w3306, "VISA Refnum in"=w3307) -> ()  [unwired: 10 in]
                          }
                          frame #1 {
                            n2856 = local read "VISA Refnum in\nfor Pump"() -> (w3308:refnum<visa-resource-name>)
                            n2857 = call "ProcessCompletionWaiter (SubVI).vi"("VISA Refnum in"=w3308) -> ()  [unwired: 11 in]
                          }
                          frame #2 {
                            n2858 = local read "VISA Refnum in\nfor Valve"() -> (w3312:refnum<visa-resource-name>)
                            n2859 = local read "External Valve \nOPEN"() -> (w3313:string)
                            n2860 = local write "Valve V3 Open"(FALSE ("Valve V3 Open")) -> ()
                            n2861 = local write "Valve V4 Open"(FALSE ("Valve V4 Open")) -> ()
                            n2862 = local write "Valve V1 Open"(TRUE ("Valve V1 Open")) -> ()
                            n2863 = local write "Valve V2 Open"(TRUE ("Valve V2 Open")) -> ()
                            n2864 = call "PortChanger_Valve (SubVI).vi"("Port Number"=w3313, "VISA Refnum in"=w3312) -> ()  [unwired: 10 in]
                            n2865 = local write "Valve V5 Open"(FALSE ("Valve V5 Open")) -> ()
                            n2866 = local write "Valve V6 Open"(FALSE ("Valve V6 Open")) -> ()
                            n2867 = local write "Valve V7 Open"(FALSE ("Valve V7 Open")) -> ()
                          }
                          frame #3 {
                            n2868 = local read "Buffer-A2 Volume \nto be Pumped"() -> (w3321:dbl)
                            n2869 = local read "Apparent Volume\nof Syringe"() -> (w3318:dbl)
                            n2870 = Quotient & Remainder(x=w3321, y=w3318) -> (x-y*floor(x/y)=w3319:dbl, floor(x/y)=w3320:dbl)
                            n2871 = for {
                              N: w3320 -> [_]
                              n2872 = stacked-sequence {
                                frame #0 {
                                n2873 = local read "Buffer-A2 PickUp \nFlow Rate (ul/min)"() -> (w3324:dbl)
                                n2874 = local read "Buffer-A2 Pumping\nResolution"() -> (w3323:T2)
                                n2875 = local read "VISA Refnum in\nfor Pump"() -> (w3326:refnum<visa-resource-name>)
                                n2876 = local read "Apparent Volume\nof Syringe"() -> (w3322:dbl)
                                n2877 = local read "Volume of Syringe"() -> (w3325:dbl)
                                n2878 = call "RPickUp(SubVI).vi"("Volume to be picked up"=w3322, "Volume of Syringe"=w3325, "Resolution of PickUP"=w3323, "PickUp Flow Rate (ul/min)"=w3324, "VISA Refnum in"=w3326) -> ()  [unwired: 6 in, 1 out]
                                }
                                frame #1 {
                                n2879 = local read "Stopper that ends \nthe main loops"() -> (w3327:bool)
                                n2880 = local read "VISA Refnum in\nfor Pump"() -> (w3328:refnum<visa-resource-name>)
                                n2881 = case shown="True" w3327 {
                                frame False {
                                }
                                frame True {
                                n2882 = local read "VISA Refnum in\nfor Pump"() -> (w3329:refnum<visa-resource-name>)
                                n2883 = call "HardStopCurrentProcess (SubVI).vi"("VISA Refnum in"=w3329) -> ()  [unwired: 11 in]
                                }
                                }
                                n2884 = call "ProcessCompletionWaiter (SubVI).vi"("VISA Refnum in"=w3328) -> ()  [unwired: 11 in]
                                }
                                frame #2 {
                                # "Reads the initial Plunger Position for computing the volume dispensed"
                                n2885 = local read "VISA Refnum in\nfor Pump"() -> (w3331:refnum<visa-resource-name>)
                                n2886 = call "AbsolutePlungerPosition (SubVI).vi"("VISA Refnum in"=w3331) -> ("Plunger Position"=w3330:i32)  [unwired: 10 in]
                                n2887 = local write "Initial Plunger Position"(w3330) -> ()
                                }
                                frame #3 {
                                # "Switch to Port-2"
                                # "Port-2 of the pump is conncted to column-1 of chip"
                                n2888 = local read "VISA Refnum in\nfor Pump"() -> (w3333:refnum<visa-resource-name>)
                                n2889 = call "PortChanger (SubVI).vi"("Port Number"="2", "VISA Refnum in"=w3333) -> ()  [unwired: 10 in]
                                }
                                frame #4 {
                                n2890 = local read "Stopper that ends \nthe main loops"() -> (w3334:bool)
                                n2891 = local read "VISA Refnum in\nfor Pump"() -> (w3335:refnum<visa-resource-name>)
                                n2892 = case shown="True" w3334 {
                                frame False {
                                }
                                frame True {
                                n2893 = local read "VISA Refnum in\nfor Pump"() -> (w3336:refnum<visa-resource-name>)
                                n2894 = call "HardStopCurrentProcess (SubVI).vi"("VISA Refnum in"=w3336) -> ()  [unwired: 11 in]
                                }
                                }
                                n2895 = call "ProcessCompletionWaiter (SubVI).vi"("VISA Refnum in"=w3335) -> ()  [unwired: 11 in]
                                }
                                frame #5 {
                                # "Keeps the AMF valve after column-1 open and valve after column-2 closed"
                                n2896 = local read "Buffer-A2 Dispense\nFlow Rate (ul/min)"() -> (w3340:dbl)
                                n2897 = local read "Buffer-A2 Pumping\nResolution"() -> (w3339:T2)
                                n2898 = local read "VISA Refnum in\nfor Pump"() -> (w3342:refnum<visa-resource-name>)
                                n2899 = local write "Pause Data Collection"(FALSE ("Pause Data Collection")) -> ()
                                n2900 = local read "Volume of Syringe"() -> (w3341:dbl)
                                n2901 = call "GoToAbsolutePosition(SubVI).vi"("Absolute Volume Position in Syringe (in ul)"=0.0 ("Volume to be Dispensed"), "Volume of Syringe"=w3341, "Resolution of Pumping"=w3339, "Flow Rate (ul/min)"=w3340, "VISA Refnum in"=w3342) -> ()  [unwired: 6 in, 1 out]
                                }
                                frame #6 {
                                n2902 = local read "Buffer-A2 Pumping\nResolution"() -> (w3344:T2)
                                n2903 = local read "VISA Refnum in\nfor Pump"() -> (w3346:refnum<visa-resource-name>)
                                n2904 = local read "Initial Plunger Position"() -> (w3345:dbl)
                                n2905 = local read "Volume of Syringe"() -> (w3343:dbl)
                                n2906 = while {
                                tunnel: w3345 -> [w3353]
                                tunnel: w3346 -> [w3352]
                                tunnel: w3344 -> [w3351]
                                tunnel: w3343 -> [w3350]
                                stop <- w3348 stop-if-true
                                n2907 = stacked-sequence {
                                tunnel: w3353 -> [w3360 _]
                                tunnel: w3352 -> [w3359 w3380]
                                tunnel: w3351 -> [w3358 _]
                                tunnel: w3350 -> [w3357 _]
                                tunnel: [_ w3378] -> w3348
                                frame #0 {
                                n2908 = call "AbsolutePlungerPosition (SubVI).vi"("VISA Refnum in"=w3359) -> ("Plunger Position"=w3356:i32)  [unwired: 10 in]
                                n2909 = case shown="\"Standard Pumping\", Default" w3358 {
                                tunnel: w3360 -> [w3365 w3374]
                                tunnel: w3356 -> [w3366 w3373]
                                tunnel: [w3364 w3371] -> w3355
                                tunnel: w3357 -> [w3363 w3372]
                                frame "Standard Pumping", Default {
                                n2910 = Subtract(x=w3365, y=w3366) -> (x-y=w3362:dbl)
                                n2911 = Absolute Value(x=w3362) -> (abs(x)=w3361:dbl)
                                n2912 = Multiply(x=w3361, y=w3363) -> (x*y=w3368:dbl)
                                n2913 = Divide(x=w3368, y=3000.0) -> (x/y=w3364:dbl)
                                }
                                frame "High Resolution Pumping" {
                                n2914 = Subtract(x=w3374, y=w3373) -> (x-y=w3370:dbl)
                                n2915 = Absolute Value(x=w3370) -> (abs(x)=w3369:dbl)
                                n2916 = Multiply(x=w3369, y=w3372) -> (x*y=w3376:dbl)
                                n2917 = Divide(x=w3376, y=24000.0) -> (x/y=w3371:dbl)
                                }
                                }
                                n2918 = local write "Volume being Injected \nin this process"(w3355) -> ()
                                }
                                frame #1 {
                                n2919 = call "LSPOneStatus (SubVI).vi"("VISA Refnum in"=w3380) -> ("read buffer"=w3382:string)  [unwired: 10 in]
                                n2920 = call <vilib>:"Trim Whitespace.vi"("string"=w3382) -> ("trimmed string"=w3381:string)  [unwired: 1 in]
                                n2921 = local read "Stopper that ends \nthe main loops"() -> (w3377:bool)
                                n2922 = Equal?(x=w3381, y="/0`\u0003") -> (x = y?=w3379:bool)
                                n2923 = Or(x=w3379, y=w3377) -> (x .or. y?=w3378:bool)
                                }
                                }
                                n2924 = Wait (ms)(milliseconds to wait=u32 100) -> ()  [unwired: 1 out]
                                n2925 = local read "Stopper that ends \nthe main loops"() -> (w3347:bool)
                                n2926 = case shown="True" w3347 {
                                frame False {
                                }
                                frame True {
                                n2927 = local read "VISA Refnum in\nfor Pump"() -> (w3354:refnum<visa-resource-name>)
                                n2928 = call "HardStopCurrentProcess (SubVI).vi"("VISA Refnum in"=w3354) -> ()  [unwired: 11 in]
                                }
                                }
                                }
                                }
                                frame #7 {
                                # "Change the port back to Buffer-A2"
                                n2929 = local read "VISA Refnum in\nfor Pump"() -> (w3385:refnum<visa-resource-name>)
                                n2930 = local read "Port for \nA2-Wash"() -> (w3384:string)
                                n2931 = local write "Pause Data Collection"(TRUE ("Pause Data Collection")) -> ()
                                n2932 = Wait (ms)(milliseconds to wait=u32 500) -> ()  [unwired: 1 out]
                                n2933 = call "PortChanger (SubVI).vi"("Port Number"=w3384, "VISA Refnum in"=w3385) -> ()  [unwired: 10 in]
                                }
                                frame #8 {
                                n2934 = local read "VISA Refnum in\nfor Pump"() -> (w3388:refnum<visa-resource-name>)
                                n2935 = local write "Volume being Injected \nin this process"(0.0 ("Volume being Injected \nin this process")) -> ()
                                n2936 = call "ProcessCompletionWaiter (SubVI).vi"("VISA Refnum in"=w3388) -> ()  [unwired: 11 in]
                                }
                              }
                            }
                            n2937 = local write "Reminder of the \nVolume to be \nPumped"(w3319) -> ()
                          }
                          frame #4 {
                            n2938 = stacked-sequence {
                              frame #0 {
                                n2939 = local read "Buffer-A2 PickUp \nFlow Rate (ul/min)"() -> (w3392:dbl)
                                n2940 = local read "Buffer-A2 Pumping\nResolution"() -> (w3391:T2)
                                n2941 = local read "VISA Refnum in\nfor Pump"() -> (w3394:refnum<visa-resource-name>)
                                n2942 = local read "Reminder of the \nVolume to be \nPumped"() -> (w3390:dbl)
                                n2943 = local read "Volume of Syringe"() -> (w3393:dbl)
                                n2944 = call "RPickUp(SubVI).vi"("Volume to be picked up"=w3390, "Volume of Syringe"=w3393, "Resolution of PickUP"=w3391, "PickUp Flow Rate (ul/min)"=w3392, "VISA Refnum in"=w3394) -> ()  [unwired: 6 in, 1 out]
                              }
                              frame #1 {
                                n2945 = local read "Stopper that ends \nthe main loops"() -> (w3395:bool)
                                n2946 = local read "VISA Refnum in\nfor Pump"() -> (w3396:refnum<visa-resource-name>)
                                n2947 = case shown="True" w3395 {
                                frame False {
                                }
                                frame True {
                                n2948 = local read "VISA Refnum in\nfor Pump"() -> (w3397:refnum<visa-resource-name>)
                                n2949 = call "HardStopCurrentProcess (SubVI).vi"("VISA Refnum in"=w3397) -> ()  [unwired: 11 in]
                                }
                                }
                                n2950 = call "ProcessCompletionWaiter (SubVI).vi"("VISA Refnum in"=w3396) -> ()  [unwired: 11 in]
                              }
                              frame #2 {
                                # "Reads the initial Plunger Position for computing the volume dispensed"
                                n2951 = local read "VISA Refnum in\nfor Pump"() -> (w3399:refnum<visa-resource-name>)
                                n2952 = call "AbsolutePlungerPosition (SubVI).vi"("VISA Refnum in"=w3399) -> ("Plunger Position"=w3398:i32)  [unwired: 10 in]
                                n2953 = local write "Initial Plunger Position"(w3398) -> ()
                              }
                              frame #3 {
                                # "Switch to Port-2"
                                # "Port-2 of the pump is conncted to column-1 of chip"
                                n2954 = local read "VISA Refnum in\nfor Pump"() -> (w3401:refnum<visa-resource-name>)
                                n2955 = call "PortChanger (SubVI).vi"("Port Number"="2", "VISA Refnum in"=w3401) -> ()  [unwired: 10 in]
                              }
                              frame #4 {
                                n2956 = local read "Stopper that ends \nthe main loops"() -> (w3402:bool)
                                n2957 = local read "VISA Refnum in\nfor Pump"() -> (w3403:refnum<visa-resource-name>)
                                n2958 = case shown="True" w3402 {
                                frame False {
                                }
                                frame True {
                                n2959 = local read "VISA Refnum in\nfor Pump"() -> (w3404:refnum<visa-resource-name>)
                                n2960 = call "HardStopCurrentProcess (SubVI).vi"("VISA Refnum in"=w3404) -> ()  [unwired: 11 in]
                                }
                                }
                                n2961 = call "ProcessCompletionWaiter (SubVI).vi"("VISA Refnum in"=w3403) -> ()  [unwired: 11 in]
                              }
                              frame #5 {
                                # "Keeps the AMF valve after column-1 open and valve after column-2 closed"
                                n2962 = local read "Buffer-A2 Dispense\nFlow Rate (ul/min)"() -> (w3408:dbl)
                                n2963 = local read "Buffer-A2 Pumping\nResolution"() -> (w3407:T2)
                                n2964 = local read "VISA Refnum in\nfor Pump"() -> (w3410:refnum<visa-resource-name>)
                                n2965 = local write "Pause Data Collection"(FALSE ("Pause Data Collection")) -> ()
                                n2966 = local read "Volume of Syringe"() -> (w3409:dbl)
                                n2967 = call "GoToAbsolutePosition(SubVI).vi"("Absolute Volume Position in Syringe (in ul)"=0.0 ("Volume to be Dispensed"), "Volume of Syringe"=w3409, "Resolution of Pumping"=w3407, "Flow Rate (ul/min)"=w3408, "VISA Refnum in"=w3410) -> ()  [unwired: 6 in, 1 out]
                              }
                              frame #6 {
                                n2968 = local read "Buffer-A2 Pumping\nResolution"() -> (w3412:T2)
                                n2969 = local read "VISA Refnum in\nfor Pump"() -> (w3414:refnum<visa-resource-name>)
                                n2970 = local read "Initial Plunger Position"() -> (w3413:dbl)
                                n2971 = local read "Volume of Syringe"() -> (w3411:dbl)
                                n2972 = while {
                                tunnel: w3413 -> [w3421]
                                tunnel: w3414 -> [w3420]
                                tunnel: w3412 -> [w3419]
                                tunnel: w3411 -> [w3418]
                                stop <- w3416 stop-if-true
                                n2973 = stacked-sequence {
                                tunnel: w3421 -> [w3428 _]
                                tunnel: w3420 -> [w3427 w3448]
                                tunnel: w3419 -> [w3426 _]
                                tunnel: w3418 -> [w3425 _]
                                tunnel: [_ w3446] -> w3416
                                frame #0 {
                                n2974 = call "AbsolutePlungerPosition (SubVI).vi"("VISA Refnum in"=w3427) -> ("Plunger Position"=w3424:i32)  [unwired: 10 in]
                                n2975 = case shown="\"Standard Pumping\", Default" w3426 {
                                tunnel: w3428 -> [w3433 w3442]
                                tunnel: w3424 -> [w3434 w3441]
                                tunnel: [w3432 w3439] -> w3423
                                tunnel: w3425 -> [w3431 w3440]
                                frame "Standard Pumping", Default {
                                n2976 = Subtract(x=w3433, y=w3434) -> (x-y=w3430:dbl)
                                n2977 = Absolute Value(x=w3430) -> (abs(x)=w3429:dbl)
                                n2978 = Multiply(x=w3429, y=w3431) -> (x*y=w3436:dbl)
                                n2979 = Divide(x=w3436, y=3000.0) -> (x/y=w3432:dbl)
                                }
                                frame "High Resolution Pumping" {
                                n2980 = Subtract(x=w3442, y=w3441) -> (x-y=w3438:dbl)
                                n2981 = Absolute Value(x=w3438) -> (abs(x)=w3437:dbl)
                                n2982 = Multiply(x=w3437, y=w3440) -> (x*y=w3444:dbl)
                                n2983 = Divide(x=w3444, y=24000.0) -> (x/y=w3439:dbl)
                                }
                                }
                                n2984 = local write "Volume being Injected \nin this process"(w3423) -> ()
                                }
                                frame #1 {
                                n2985 = call "LSPOneStatus (SubVI).vi"("VISA Refnum in"=w3448) -> ("read buffer"=w3450:string)  [unwired: 10 in]
                                n2986 = call <vilib>:"Trim Whitespace.vi"("string"=w3450) -> ("trimmed string"=w3449:string)  [unwired: 1 in]
                                n2987 = local read "Stopper that ends \nthe main loops"() -> (w3445:bool)
                                n2988 = Equal?(x=w3449, y="/0`\u0003") -> (x = y?=w3447:bool)
                                n2989 = Or(x=w3447, y=w3445) -> (x .or. y?=w3446:bool)
                                }
                                }
                                n2990 = Wait (ms)(milliseconds to wait=u32 100) -> ()  [unwired: 1 out]
                                n2991 = local read "Stopper that ends \nthe main loops"() -> (w3415:bool)
                                n2992 = case shown="True" w3415 {
                                frame False {
                                }
                                frame True {
                                n2993 = local read "VISA Refnum in\nfor Pump"() -> (w3422:refnum<visa-resource-name>)
                                n2994 = call "HardStopCurrentProcess (SubVI).vi"("VISA Refnum in"=w3422) -> ()  [unwired: 11 in]
                                }
                                }
                                }
                              }
                              frame #7 {
                                n2995 = local write "Pause Data Collection"(TRUE ("Pause Data Collection")) -> ()
                                n2996 = Wait (ms)(milliseconds to wait=u32 500) -> ()  [unwired: 1 out]
                              }
                              frame #8 {
                                n2997 = local write "Volume being Injected \nin this process"(0.0 ("Volume being Injected \nin this process")) -> ()
                                n2998 = local write "Start the Process"(FALSE ("Start the Process")) -> ()
                              }
                            }
                          }
                        }
                        n2999 = local write "Sample pumping \ninto Column-1"(FALSE ("Sample pumping \ninto Column-1")) -> ()
                        n3000 = local write "Washing Column-1"(TRUE ("Washing Column-1")) -> ()
                      }
                      frame #3 {
                        # "Connecting Buffer-C with port-5, cleaning the tubing with Buffer-C1, and washing the Column-2 to get rid of spill out from wash steps of column-1"
                        n3001 = stacked-sequence {
                          frame #0 {
                            # "Switch to Port-5"
                            # "Port-5 of pump is connected to Buffer-C1"
                            n3002 = local read "VISA Refnum in\nfor Pump"() -> (w3459:refnum<visa-resource-name>)
                            n3003 = local read "Port for \nC1-Equilibriation"() -> (w3458:string)
                            n3004 = call "PortChanger (SubVI).vi"("Port Number"=w3458, "VISA Refnum in"=w3459) -> ()  [unwired: 10 in]
                          }
                          frame #1 {
                            n3005 = local read "VISA Refnum in\nfor Pump"() -> (w3460:refnum<visa-resource-name>)
                            n3006 = call "ProcessCompletionWaiter (SubVI).vi"("VISA Refnum in"=w3460) -> ()  [unwired: 11 in]
                          }
                          frame #2 {
                            # "Wash the inside of the pump valve"
                            n3007 = local read "n"() -> (w3461:i32)
                            n3008 = for {
                              N: w3461 -> [_]
                              n3009 = stacked-sequence {
                                frame #0 {
                                n3010 = local read "Buffer-A2 Pumping\nResolution"() -> (w3464:T2)
                                n3011 = local read "VISA Refnum in\nfor Pump"() -> (w3466:refnum<visa-resource-name>)
                                n3012 = local read "V-S"() -> (w3462:dbl)
                                n3013 = local read "Volume of Syringe"() -> (w3465:dbl)
                                n3014 = call "RPickUp(SubVI).vi"("Volume to be picked up"=w3462, "Volume of Syringe"=w3465, "Resolution of PickUP"=w3464, "PickUp Flow Rate (ul/min)"=150.0, "VISA Refnum in"=w3466) -> ()  [unwired: 6 in, 1 out]
                                }
                                frame #1 {
                                n3015 = local read "Stopper that ends \nthe main loops"() -> (w3467:bool)
                                n3016 = local read "VISA Refnum in\nfor Pump"() -> (w3468:refnum<visa-resource-name>)
                                n3017 = case shown="True" w3467 {
                                frame False {
                                }
                                frame True {
                                n3018 = local read "VISA Refnum in\nfor Pump"() -> (w3469:refnum<visa-resource-name>)
                                n3019 = call "HardStopCurrentProcess (SubVI).vi"("VISA Refnum in"=w3469) -> ()  [unwired: 11 in]
                                }
                                }
                                n3020 = call "ProcessCompletionWaiter (SubVI).vi"("VISA Refnum in"=w3468) -> ()  [unwired: 11 in]
                                }
                                frame #2 {
                                # "Switch to Port-1"
                                # "Port-1 of the pump is conncted to waste"
                                n3021 = local read "VISA Refnum in\nfor Pump"() -> (w3471:refnum<visa-resource-name>)
                                n3022 = call "PortChanger (SubVI).vi"("Port Number"="1", "VISA Refnum in"=w3471) -> ()  [unwired: 10 in]
                                }
                                frame #3 {
                                n3023 = local read "Stopper that ends \nthe main loops"() -> (w3472:bool)
                                n3024 = local read "VISA Refnum in\nfor Pump"() -> (w3473:refnum<visa-resource-name>)
                                n3025 = case shown="True" w3472 {
                                frame False {
                                }
                                frame True {
                                n3026 = local read "VISA Refnum in\nfor Pump"() -> (w3474:refnum<visa-resource-name>)
                                n3027 = call "HardStopCurrentProcess (SubVI).vi"("VISA Refnum in"=w3474) -> ()  [unwired: 11 in]
                                }
                                }
                                n3028 = call "ProcessCompletionWaiter (SubVI).vi"("VISA Refnum in"=w3473) -> ()  [unwired: 11 in]
                                }
                                frame #4 {
                                n3029 = local read "Buffer-A2 Pumping\nResolution"() -> (w3477:T2)
                                n3030 = local read "VISA Refnum in\nfor Pump"() -> (w3479:refnum<visa-resource-name>)
                                n3031 = local read "Volume of Syringe"() -> (w3478:dbl)
                                n3032 = call "GoToAbsolutePosition(SubVI).vi"("Absolute Volume Position in Syringe (in ul)"=0.0 ("Volume to be Dispensed"), "Volume of Syringe"=w3478, "Resolution of Pumping"=w3477, "Flow Rate (ul/min)"=150.0, "VISA Refnum in"=w3479) -> ()  [unwired: 6 in, 1 out]
                                }
                                frame #5 {
                                n3033 = local read "VISA Refnum in\nfor Pump"() -> (w3480:refnum<visa-resource-name>)
                                n3034 = call "ProcessCompletionWaiter (SubVI).vi"("VISA Refnum in"=w3480) -> ()  [unwired: 11 in]
                                }
                                frame #6 {
                                # "Change the port back to Buffer-C1"
                                n3035 = local read "VISA Refnum in\nfor Pump"() -> (w3482:refnum<visa-resource-name>)
                                n3036 = local read "Port for \nC1-Equilibriation"() -> (w3481:string)
